vi "toVariant.vi"(8 "error in (no error)":errorcluster, 11 "VariantMessage in":refnum<class "VariantMessage.lvclass">) -> (0 "error out":errorcluster, 1 "Variant":variant, 2 "Type":i32, 3 "VariantMessage out":refnum<class "VariantMessage.lvclass">)   [LabVIEW 2013, in "VariantMessage.lvclass"]
doc: "Formats the message to a application specific type integer and a variant.\n\nMessages that are of variant type can be used to send messages to the driver itself. The driver will examine all incoming messages and any variant type messages will be interpreted according to the type integer"
uses:
  VariantMessage.lvclass
  VariantMessage.lvclass/VariantMessage.ctl
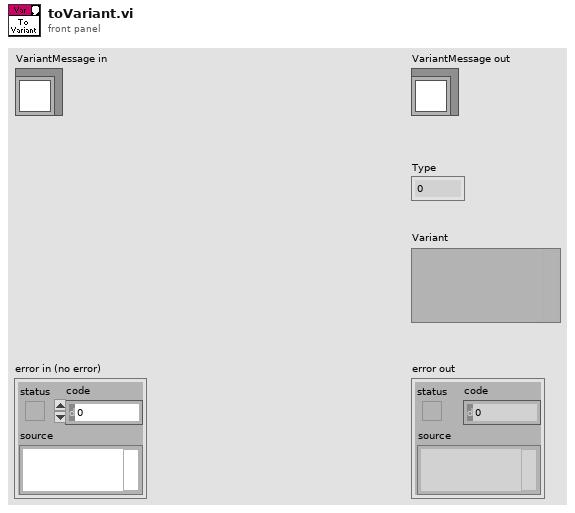
[diagram p1: front panel]
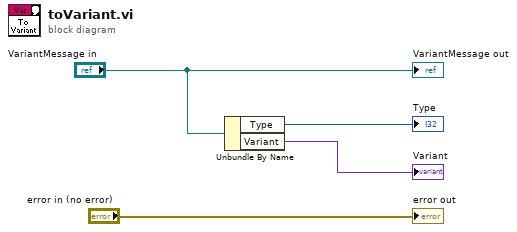
[diagram p0: block diagram]
diagram:
  n1 = Unbundle By Name("VariantMessage in") -> ("Type"=→"Type":i32, "Variant"=→"Variant":variant)
  "error out" <- "error in (no error)"
  "VariantMessage out" <- "VariantMessage in"
